vi "RunTest.vi"(8 "error in":errorcluster, 11 "Prueba21 in":refnum<class "Prueba21.lvclass">) -> (0 "error out":errorcluster, 2 "Resultado":string, 3 "Prueba21 out":refnum<class "Prueba21.lvclass">)   [LabVIEW 2019, in "Prueba21.lvclass"]
uses:
  Prueba21.lvclass
  Prueba21.lvclass/Prueba21.ctl
  QMH/Message Queue/Enqueue Message (Single).vi
  <vilib>/Utility/error.llb/Error Cluster From Error Code.vi
  RerenceAllControlsToolkit/_get mutiple control reference by name.vi
  RerenceAllControlsToolkit/_get control reference by name.vi
  <vilib>/ErrorRing/Error Ring.xnode
  QMH/Message Queue/Message Queue.lvlib
  QMH/User Event - Stop/User Event - Stop.lvlib
  Prueba/Prueba.lvclass
panel:
  out "TD":dbl
  out "Frecuencia":dbl
  out "voltaje":dbl
  in  "generar_ext":bool
  in  "Tab Control":enum32{"D1", "D2"}(tab)
  in  "CapturaGlobal_D1":bool
  in  "3_D1":bool
  in  "2_D1":bool
  out "LedVerdeD1":bool=TRUE
  in  "1_D1":bool
  out "LedRojoD1":bool=TRUE
  in  "Capturar_D1":bool
  out "Tabla_Referencia":string[][](table)
  out "grafica_frec_1":cluster{"f0":dbl, "df":dbl, "magnitude":dbl[]}[](graph) caption="Presion Sonora Vs Frencuencia"
  out "grafica_tiempo_1":waveform(dbl)[](graph) caption="Presion Sonora Vs Tiempo"
  in  "seguir_D2":bool
  in  "Capturar_D2":bool
  out "LedRojoD2":bool=TRUE
  out "LedVerdeD2":bool=TRUE
  in  "1_D2":bool
  in  "2_D2":bool
  in  "3_D2":bool
  out "Tabla_Presion_Sonora":string[][](table)
  out "Tabla_Frecuencia":string[][](table)
  out "Tabla_Distorsion_Total":string[][](table)
  out "grafica_frec_2":cluster{"f0":dbl, "df":dbl, "magnitude":dbl[]}[](graph) caption="Presion Sonora Vs Frencuencia"
  out "grafica_tiempo_2":waveform(dbl)[](graph) caption="Presion Sonora Vs Tiempo."
  in  "CapturaGlobal_D2":bool
  out "cumple":bool
  out "no_cumple":bool
  in  "salir":bool
  # "Captura Individual"
  # "21. Medición Nivel de Presión Sonora Calibrador Patrón"
  # "Nivel de Presión Sonora"
  # "Frecuencia"
  # "Distorsión Total (TD)"
  # "Captura Individual"
  # "Cumple"
  # "No Cumple"
  # "21. Medición Nivel de Presión Sonora Calibrador Patrón"
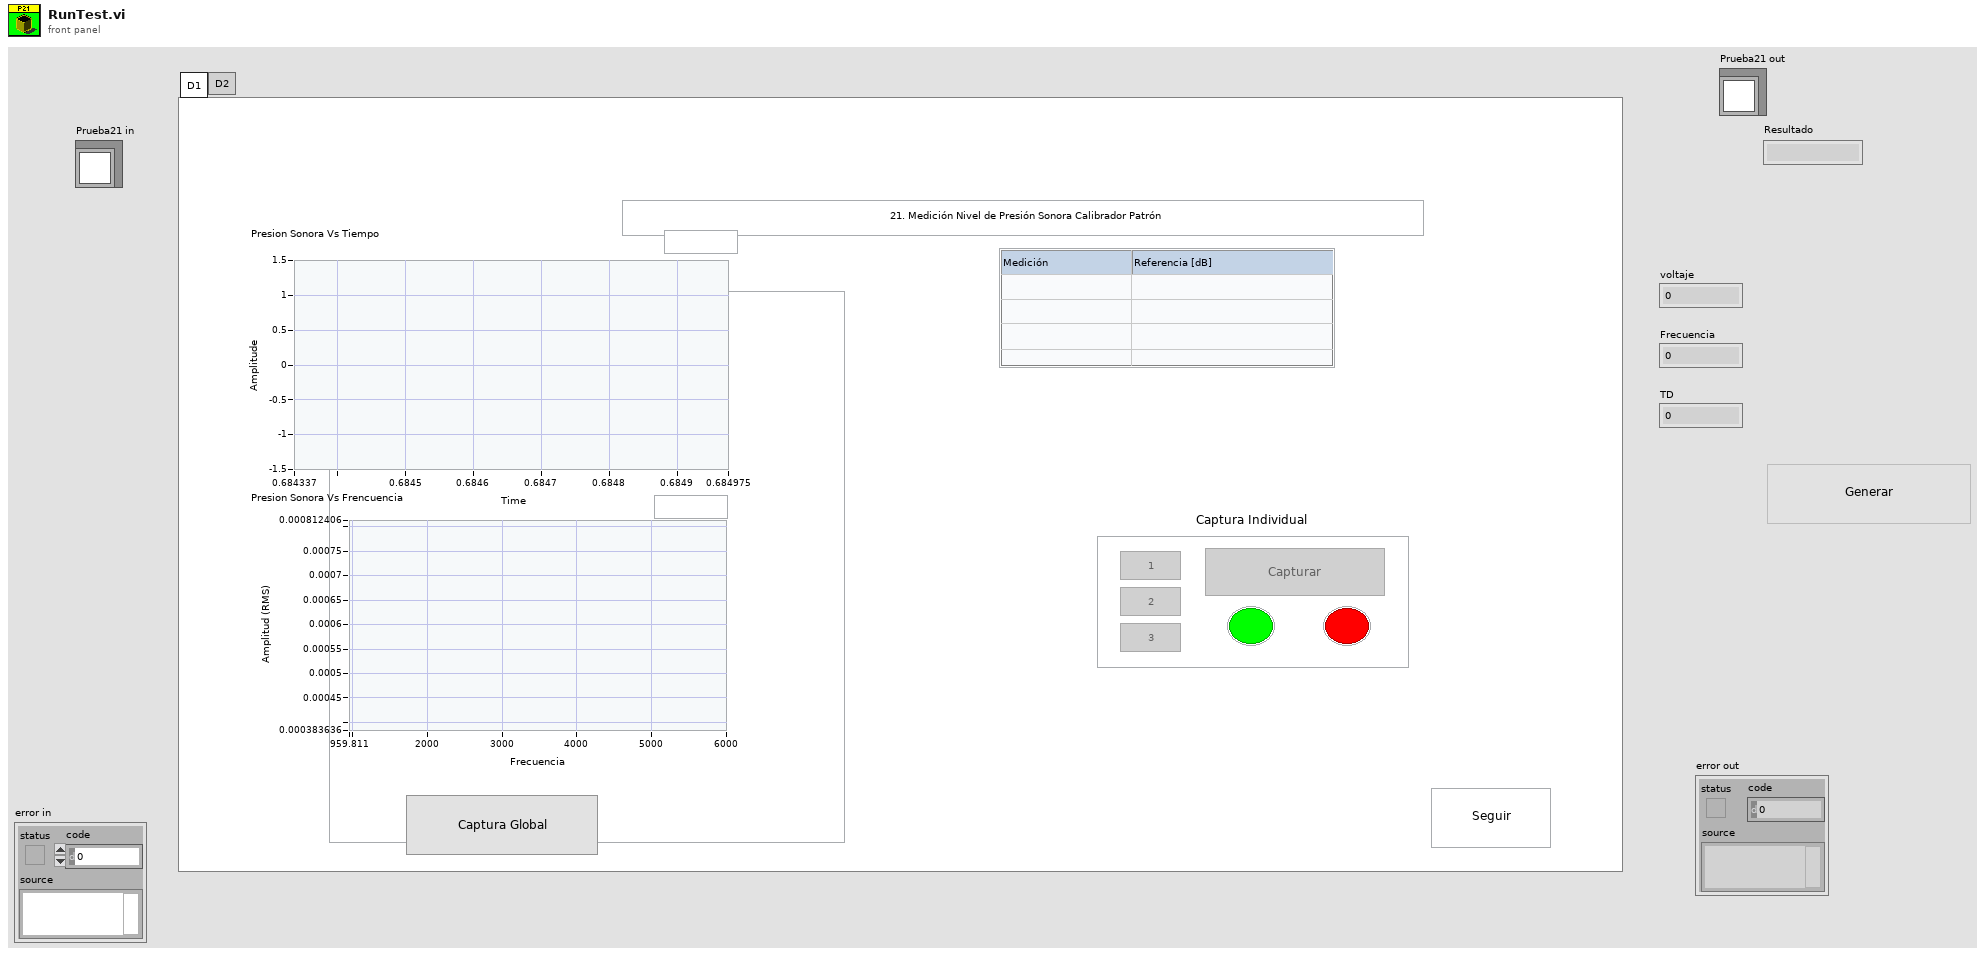
[diagram p1: front panel]
types:
  T1 = typedef "Message Queue.lvlib/All Message Queues.ctl" = cluster{"MHL":refnum<queue>, "Inst_CNT90":refnum<queue>, "Inst_DS360":refnum<queue>, "Inst_Keithley2002":refnum<queue>, "Inst_DAQ":refnum<queue>, "BD":refnum<queue>, "Pistofono":refnum<queue>, "Nexus":refnum<queue>}
  T2 = cluster{"ControlName":string, "ControlReference":refnum<vi>}[]
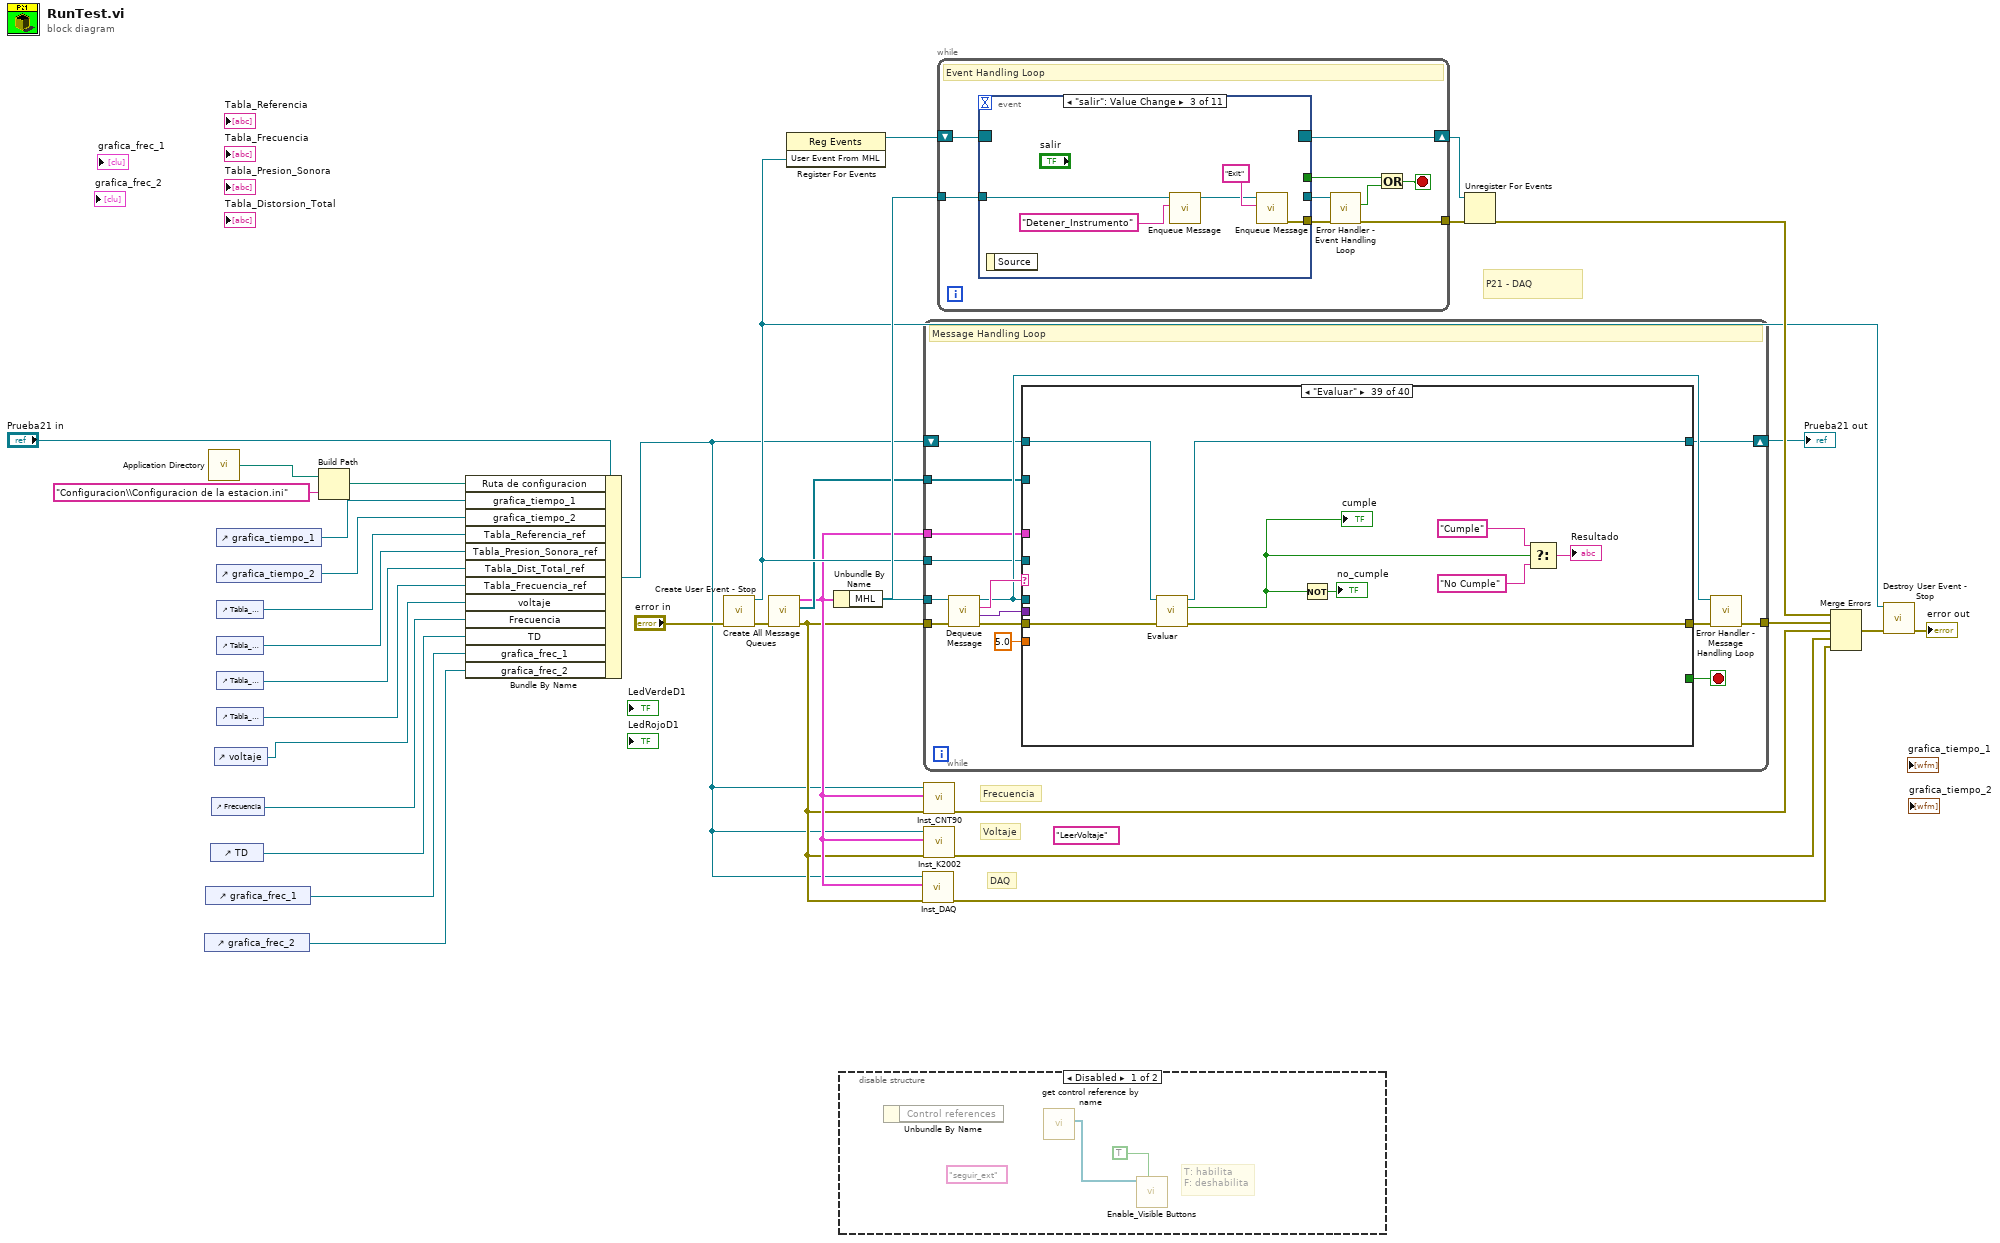
[diagram p0: block diagram]
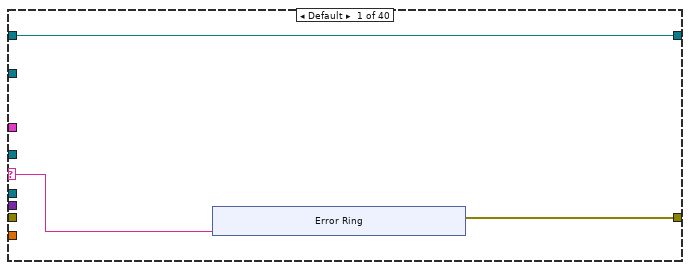
[diagram p3: hidden frame]
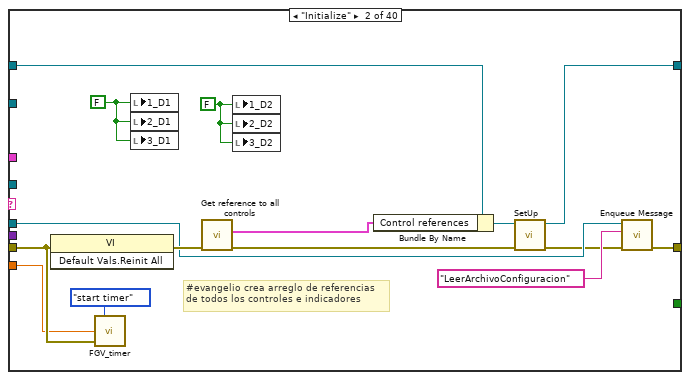
[diagram p4: hidden frame]
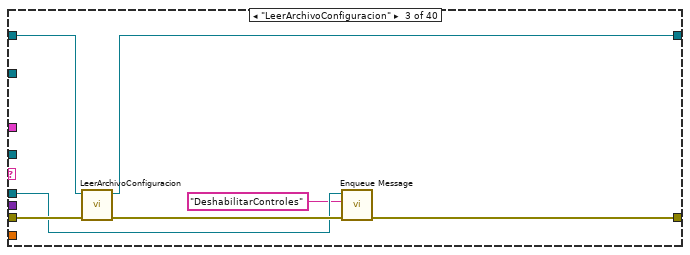
[diagram p5: hidden frame]
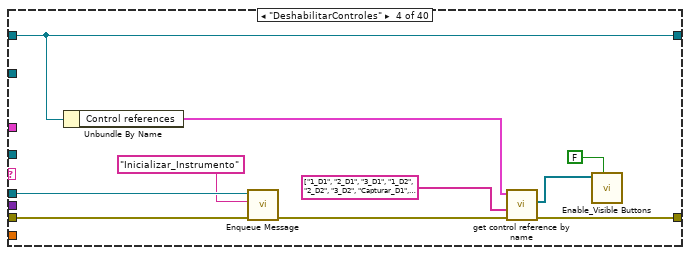
[diagram p6: hidden frame]
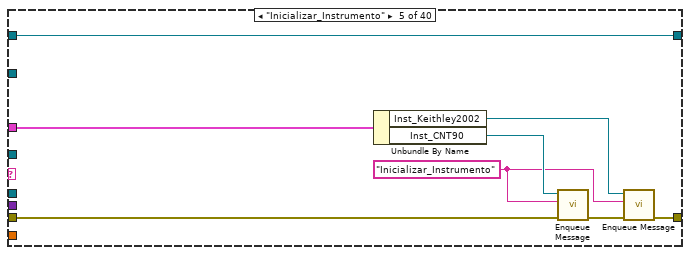
[diagram p7: hidden frame]
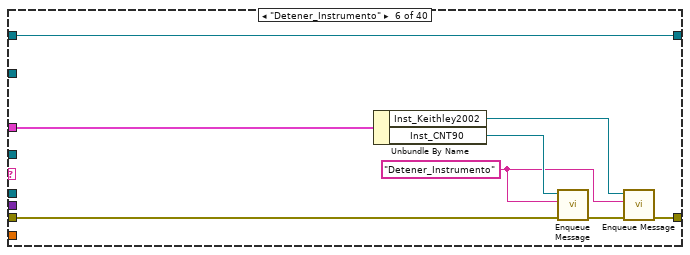
[diagram p8: hidden frame]
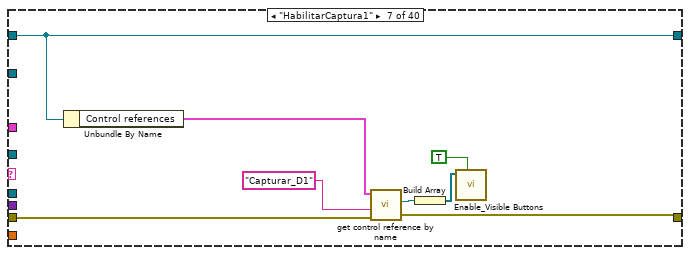
[diagram p9: hidden frame]
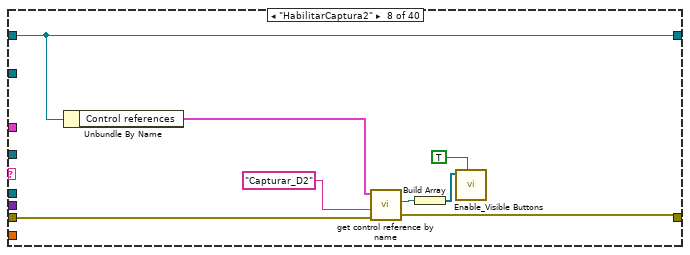
[diagram p10: hidden frame]
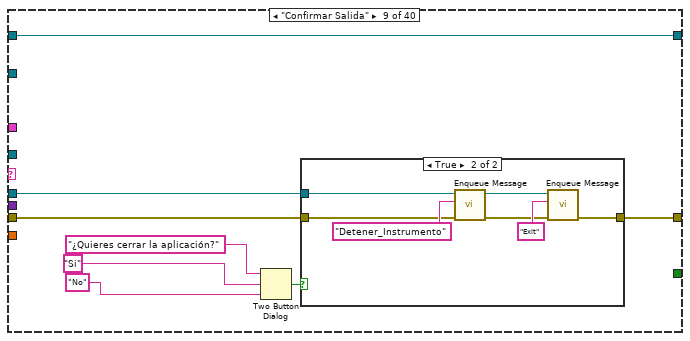
[diagram p11: hidden frame]
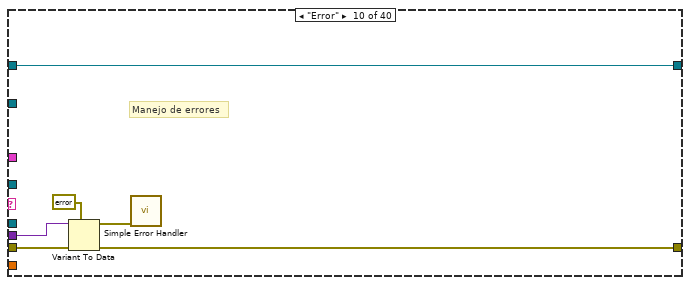
[diagram p13: hidden frame]
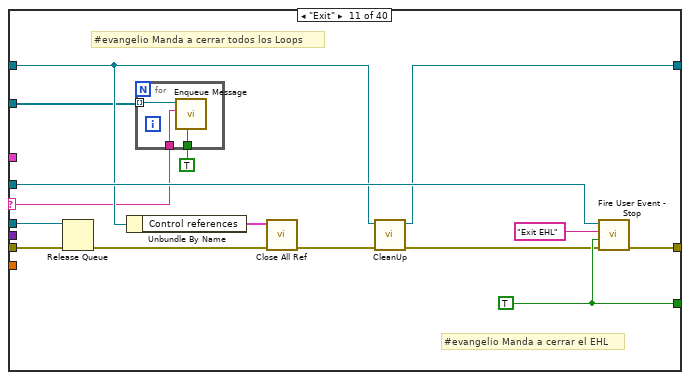
[diagram p14: hidden frame]
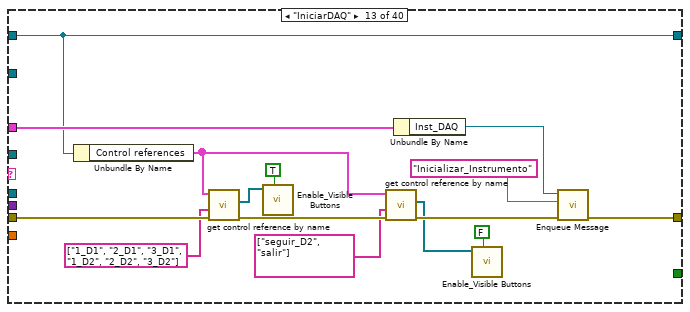
[diagram p16: hidden frame]
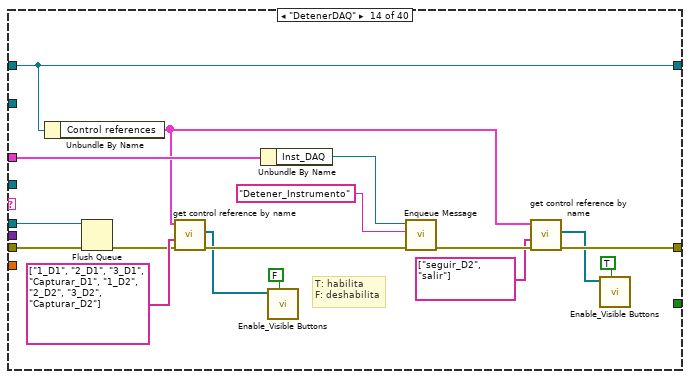
[diagram p17: hidden frame]
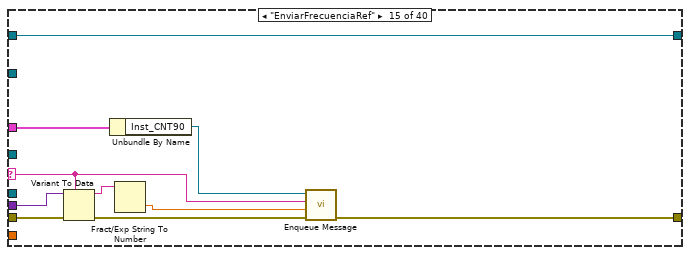
[diagram p18: hidden frame]
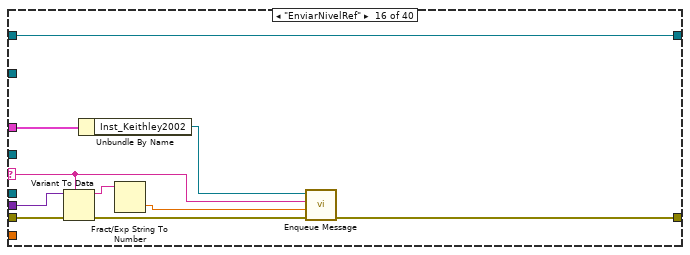
[diagram p19: hidden frame]
diagram:
  (unwired) "LeerVoltaje" ("Message")
  # "P21 - DAQ"
  # "DAQ"
  # "Voltaje"
  # "Frecuencia"
  n1 = control-ref of="grafica_frec_2"() -> (w1:refnum<vi>)
  n2 = control-ref of="grafica_frec_1"() -> (w2:refnum<vi>)
  n3 = call <vilib>:"Application Directory.vi"() -> ("Application Directory"=w19:path)
  n4 = control-ref of="TD"() -> (w3:refnum<vi>)
  n5 = control-ref of="Frecuencia"() -> (w4:refnum<vi>)
  n6 = control-ref of="voltaje"() -> (w5:refnum<vi>)
  n7 = control-ref of="grafica_tiempo_1"() -> (w12:refnum<vi>)
  n8 = control-ref of="grafica_tiempo_2"() -> (w11:refnum<vi>)
  n9 = control-ref of="Tabla_Referencia"() -> (w9:refnum<vi>)
  n10 = control-ref of="Tabla_Presion_Sonora"() -> (w8:refnum<vi>)
  n11 = control-ref of="Tabla_Distorsion_Total"() -> (w7:refnum<vi>)
  n12 = control-ref of="Tabla_Frecuencia"() -> (w6:refnum<vi>)
  n13 = Build Path(base path=w19, name or relative path="Configuracion\\Configuracion de la estacion.ini") -> (appended path=w18:path)
  n14 = Bundle By Name(cluster="Prueba21 in", "Ruta de configuracion"=w18, "grafica_tiempo_1"=w12, "grafica_tiempo_2"=w11, "Tabla_Referencia_ref"=w9, "Tabla_Presion_Sonora_ref"=w8, "Tabla_Dist_Total_ref"=w7, "Tabla_Frecuencia_ref"=w6, "voltaje"=w5, "Frecuencia"=w4, "TD"=w3, "grafica_frec_1"=w2, "grafica_frec_2"=w1) -> (w10:refnum<class "Prueba21.lvclass">)
  n15 = call "Create User Event - Stop.vi"("error in (no error)"="error in") -> ("error out"=w31:errorcluster, "User Event From MHL"=w25:refnum<user-event>)  [unwired: 9 in]
  n16 = call "Create All Message Queues.vi"("error in (no error)"=w31) -> ("error out"=w14:errorcluster, "PL Queues Array"=w16:refnum<queue>[], "All Message Queues out"=w15:T1)  [unwired: 8 in]
  n17 = register-events(w25) -> (reference out=w34:refnum<event-registration>)  [unwired: 2 in, 1 out]
  n18 = Unbundle By Name(w15) -> ("MHL"=w30:refnum<queue>)
  n19 = disable-structure shown="Disabled" {
    frame Disabled {
      (unwired) "seguir_ext" ("Control name")
      # "T: habilita\nF: deshabilita"
      n20 = Unbundle By Name() -> ("Control references"=w35)  [unwired: 1 in]
      n21 = call-poly "get control reference by name.vi"() -> ("error out"=w37:errorcluster, "References"=w36:refnum<vi>[], "Control names"=w39:string[])  [unwired: 5 in]
      n22 = call "Enable_Visible Buttons.vi"("Enable? (T)"=TRUE, "Controls Ref Array"=w36) -> ()  [unwired: 10 in]
    }
    frame Enabled {
    }
  }
  n23 = call "Inst_DAQ.vi"("error in"=w14, "All Message Queues in"=w15, "Prueba31 in"=w10) -> ("error out"=w13:errorcluster)  [unwired: 8 in]
  n24 = while {
    tunnel: w14 -> [w54]
    tunnel: w30 -> [w53]
    tunnel: [w47] -> w28
    shift-right: [w45] -> w26
    shift-left: w10 -> [w46]
    tunnel: w15 -> [w43]
    tunnel: w25 -> [w42]
    tunnel: w16 -> [w41]
    stop <- w44 stop-if-true
    # "Message Handling Loop"
    n25 = call "Dequeue Message.vi"("error in (no error)"=w54, "Message Queue"=w53) -> ("error out"=w50:errorcluster, "Message Data"=w51:variant, "Message"=w52:string, "dup Message Queue"=w49:refnum<queue>)  [unwired: 6 in]
    n26 = case shown="\"Evaluar\"" w52 {
      selector: w52 -> [w56 _ _ _ _ _ _ _ _ _ w153 _ _ _ w201 w211 _ _ _ _ _ _ _ _ _ _ _ _ _ _ _ _ _ _ _ _ _ _ _ _]
      tunnel: w49 -> [_ w76 w81 w88 _ _ _ _ w129 _ w164 _ _ w190 _ _ _ _ _ _ w254 w263 w283 w318 w332 _ _ _ _ _ w392 w403 w416 w436 w459 _ w469 _ _ _]
      tunnel: w51 -> [_ _ _ _ _ _ _ _ _ w146 _ _ _ _ w208 w218 _ _ _ _ _ _ _ _ _ _ _ _ _ _ _ _ _ w441 _ _ _ _ _ _]
      tunnel: w50 -> [_ w71 w86 w95 w97 w105 w119 w127 w135 w147 w163 w170 w178 w195 w209 w219 w222 w224 w239 w250 w259 w271 w290 w326 w335 w343 w360 w362 w377 w388 w397 w408 w424 w442 w461 w467 w478 w486 w500 w502]
      tunnel: [w55 w77 w82 w93 w99 w107 w117 w125 w134 w148 w161 w170 w175 w189 w205 w215 w222 w224 w236 w246 w257 w268 w288 w325 w334 w349 w357 w362 w374 w384 w395 w406 w421 w437 w444 w467 w470 w482 w499 w502] -> w48
      tunnel: w46 -> [w57 w78 w85 w94 w98 w106 w118 w126 w136 w150 w154 w169 w180 w196 w210 w220 w221 w223 w240 w251 w262 w267 w286 w323 w331 w342 w356 w361 w378 w389 w400 w411 w420 w439 w450 w466 w476 w484 w498 w501]
      tunnel: [w57 w66 w84 w94 w98 w106 w118 w126 w136 w150 w155 w169 w180 w196 w210 w220 w221 w223 w240 w251 w262 w265 w287 w324 w333 w342 w355 w361 w378 w389 w400 w411 w418 w439 w450 w466 w471 w483 w497 w501] -> w45
      tunnel: [_ _ _ _ _ _ _ _ _ _ w158 _ _ _ _ _ _ _ _ _ _ _ _ _ _ _ _ _ _ _ _ _ _ _ _ _ _ _ _ _] -> w44
      tunnel: w43 -> [_ _ _ _ w104 w112 _ _ _ _ _ _ w184 w200 w203 w213 _ _ w242 w245 w261 _ _ _ _ _ _ _ w380 w383 w399 w410 _ _ _ _ _ w481 _ _]
      tunnel: w42 -> [_ _ _ _ _ _ _ _ _ _ w160 _ _ _ _ _ _ _ _ _ _ _ _ _ _ _ _ _ _ _ _ _ _ _ _ _ _ _ _ _]
      tunnel: w41 -> [_ _ _ _ _ _ _ _ _ _ w151 _ _ _ _ _ _ _ _ _ _ _ _ _ _ _ _ _ _ _ _ _ _ _ _ _ _ _ _ _]
      tunnel: 5.0 ("time target") -> [_ w69 _ _ _ _ _ _ _ _ _ _ _ _ _ _ _ _ _ w248 _ w272 _ _ _ w348 _ _ _ w386 _ _ w425 _ w443 _ _ _ _ _]
      frame Default {
        n27 = xnode "Error Ring"("parameter 0"=w56) -> ("error out"=w55:errorcluster)
      }
      frame "Initialize" {
        w72 = FALSE ("1_D2")
        w73 = FALSE ("1_D1")
        # "#evangelio crea arreglo de referencias\nde todos los controles e indicadores"
        n28 = invoke class="VI" method="Default Vals.Reinit All"(error in=w71) -> (error out=w79:errorcluster)  [unwired: 2 in, 2 out]
        n29 = call "FGV_timer.vi"("error in (no error)"=w71, "time target"=w69, "action"=enum16{"get time", "start timer"}."start timer") -> ()  [unwired: 3 out]
        n30 = local write "1_D1"(w73) -> ()
        n31 = local write "2_D1"(w73) -> ()
        n32 = local write "3_D1"(w73) -> ()
        n33 = call "Get reference to all controls.vi"("error in (no error)"=w79) -> ("error out"=w67:errorcluster, "Control references"=w74:T2)  [unwired: 5 in]
        n34 = local write "1_D2"(w72) -> ()
        n35 = local write "2_D2"(w72) -> ()
        n36 = local write "3_D2"(w72) -> ()
        n37 = Bundle By Name(cluster=w78, "Control references"=w74) -> (w68:refnum<class "Prueba21.lvclass">)
        n38 = call-dynamic "SetUp.vi"("error in (no error)"=w67, "Prueba21 in"=w68) -> ("error out"=w65:errorcluster, "Prueba21 out"=w66:refnum<class "Prueba21.lvclass">)  [unwired: 8 in]
        n39 = call-poly "Enqueue Message.vi"("error in (no error)"=w65, "Message"="LeerArchivoConfiguracion", "Message Queue"=w76) -> ("error out"=w77:errorcluster)  [unwired: 7 in, 1 out]
      }
      frame "LeerArchivoConfiguracion" {
        n40 = call "LeerArchivoConfiguracion.vi"("error in"=w86, "Prueba31 in"=w85) -> ("error out"=w83:errorcluster, "Prueba31 out"=w84:refnum<class "Prueba21.lvclass">)  [unwired: 8 in]
        n41 = call-poly "Enqueue Message.vi"("error in (no error)"=w83, "Message"="DeshabilitarControles", "Message Queue"=w81) -> ("error out"=w82:errorcluster)  [unwired: 7 in, 1 out]
      }
      frame "DeshabilitarControles" {
        n42 = Unbundle By Name(w94) -> ("Control references"=w96:T2)
        n43 = call-poly "Enqueue Message.vi"("error in (no error)"=w95, "Message"="Inicializar_Instrumento", "Message Queue"=w88) -> ("error out"=w89:errorcluster)  [unwired: 7 in, 1 out]
        n44 = call-poly "get control reference by name.vi"("error in (no error)"=w89, "Control names"=string[] ["1_D1", "2_D1", "3_D1", "1_D2", "2_D2", "3_D2", "Capturar_D1", "Capturar_D2"], "Control references"=w96) -> ("error out"=w93:errorcluster, "References"=w91:refnum<vi>[])  [unwired: 3 in]
        n45 = call "Enable_Visible Buttons.vi"("Enable? (T)"=FALSE, "Controls Ref Array"=w91) -> ()  [unwired: 10 in]
      }
      frame "Inicializar_Instrumento" {
        w100 = "Inicializar_Instrumento" ("Message")
        n46 = Unbundle By Name(w104) -> ("Inst_Keithley2002"=w101:refnum<queue>, "Inst_CNT90"=w103:refnum<queue>)
        n47 = call-poly "Enqueue Message.vi"("error in (no error)"=w97, "Message"=w100, "Message Queue"=w103) -> ("error out"=w102:errorcluster)  [unwired: 7 in, 1 out]
        n48 = call-poly "Enqueue Message.vi"("error in (no error)"=w102, "Message"=w100, "Message Queue"=w101) -> ("error out"=w99:errorcluster)  [unwired: 7 in, 1 out]
      }
      frame "Detener_Instrumento" {
        w108 = "Detener_Instrumento" ("Message")
        n49 = Unbundle By Name(w112) -> ("Inst_Keithley2002"=w109:refnum<queue>, "Inst_CNT90"=w111:refnum<queue>)
        n50 = call-poly "Enqueue Message.vi"("error in (no error)"=w105, "Message"=w108, "Message Queue"=w111) -> ("error out"=w110:errorcluster)  [unwired: 7 in, 1 out]
        n51 = call-poly "Enqueue Message.vi"("error in (no error)"=w110, "Message"=w108, "Message Queue"=w109) -> ("error out"=w107:errorcluster)  [unwired: 7 in, 1 out]
      }
      frame "HabilitarCaptura1" {
        n52 = Unbundle By Name(w118) -> ("Control references"=w120:T2)
        n53 = call-poly "get control reference by name.vi"("error in (no error)"=w119, "Control name"="Capturar_D1", "Control references"=w120) -> ("error out"=w117:errorcluster, "Ctl Refnum"=w114:refnum<vi>)  [unwired: 3 in]
        n54 = Build Array(w114) -> (w113:refnum<vi>[])
        n55 = call "Enable_Visible Buttons.vi"("Enable? (T)"=TRUE, "Controls Ref Array"=w113) -> ()  [unwired: 10 in]
      }
      frame "HabilitarCaptura2" {
        n56 = Unbundle By Name(w126) -> ("Control references"=w128:T2)
        n57 = call-poly "get control reference by name.vi"("error in (no error)"=w127, "Control name"="Capturar_D2", "Control references"=w128) -> ("error out"=w125:errorcluster, "Ctl Refnum"=w122:refnum<vi>)  [unwired: 3 in]
        n58 = Build Array(w122) -> (w121:refnum<vi>[])
        n59 = call "Enable_Visible Buttons.vi"("Enable? (T)"=TRUE, "Controls Ref Array"=w121) -> ()  [unwired: 10 in]
      }
      frame "Confirmar Salida" {
        n60 = Two Button Dialog(message="¿Quieres cerrar la aplicación?", 1:"No" ("T button name (\"OK\")"), 2:"Si" ("T button name (\"OK\")")) -> (T button?=w130:bool)
        n61 = case shown="True" w130 {
          tunnel: w135 -> [w137 w140]
          tunnel: [w137 w144] -> w134
          tunnel: w129 -> [_ w141]
          frame False {
          }
          frame True {
            n62 = call-poly "Enqueue Message.vi"("error in (no error)"=w140, "Message"="Detener_Instrumento", "Message Queue"=w141) -> ("error out"=w139:errorcluster, "dup Message Queue"=w138:refnum<queue>)  [unwired: 7 in]
            n63 = call-poly "Enqueue Message.vi"("error in (no error)"=w139, "Message"="Exit", "Message Queue"=w138) -> ("error out"=w144:errorcluster)  [unwired: 7 in, 1 out]
          }
        }
      }
      frame "Error" {
        # "Manejo de errores"
        n64 = Variant To Data(error in=w147, type=errorcluster {"status"=FALSE, "code"=0, "source"=""} ("error constant"), Variant=w146) -> (data=w145:errorcluster, error out=w148:errorcluster)
        n65 = call <vilib>:"Simple Error Handler.vi"("error in (no error)"=w145) -> ()  [unwired: 4 in, 5 out]
      }
      frame "Exit" {
        w158 = TRUE
        # "#evangelio Manda a cerrar el EHL"
        # "#evangelio Manda a cerrar todos los Loops"
        n66 = Release Queue(queue=w164, error in (no error)=w163) -> (error out=w162:errorcluster)  [unwired: 1 in, 2 out]
        n67 = Unbundle By Name(w154) -> ("Control references"=w165:T2)
        n68 = for {
          tunnel: w151 -> [w168] mode=indexing
          tunnel: w153 -> [w167]
          tunnel: TRUE -> [w166]
          n69 = call-poly "Enqueue Message.vi"("Priority Message? (F)"=w166, "Message"=w167, "Message Queue"=w168) -> ()  [unwired: 7 in, 2 out]
        }
        n70 = call "Close All Ref.vi"("error in (no error)"=w162, "Control references"=w165) -> ("error out"=w157:errorcluster)  [unwired: 9 in]
        n71 = call-dynamic "CleanUp.vi"("error in (no error)"=w157, "Prueba21 in"=w154) -> ("error out"=w156:errorcluster, "Prueba21 out"=w155:refnum<class "Prueba21.lvclass">)  [unwired: 8 in]
        n72 = call "Fire User Event - Stop.vi"("error in (no error)"=w156, "Event Data"=w158, "User Event"="Exit EHL", "User Event in"=w160) -> ("error out"=w161:errorcluster)  [unwired: 7 in]
      }
      frame "---- Captura Global  ----" {
      }
      frame "IniciarDAQ" {
        n73 = Unbundle By Name(w180) -> ("Control references"=w174:T2)
        n74 = call-poly "get control reference by name.vi"("error in (no error)"=w178, "Control names"=string[] ["1_D1", "2_D1", "3_D1", "1_D2", "2_D2", "3_D2"] ("Control name"), "Control references"=w174) -> ("error out"=w179:errorcluster, "References"=w181:refnum<vi>[])  [unwired: 3 in]
        n75 = call "Enable_Visible Buttons.vi"("Enable? (T)"=TRUE, "Controls Ref Array"=w181) -> ()  [unwired: 10 in]
        n76 = call-poly "get control reference by name.vi"("Control names"=string[] ["seguir_D2", "salir"] ("Message"), "Control references"=w174) -> ("References"=w172:refnum<vi>[])  [unwired: 4 in, 1 out]
        n77 = Unbundle By Name(w184) -> ("Inst_DAQ"=w183:refnum<queue>)
        n78 = call "Enable_Visible Buttons.vi"("Enable? (T)"=FALSE, "Controls Ref Array"=w172) -> ()  [unwired: 10 in]
        n79 = call-poly "Enqueue Message.vi"("error in (no error)"=w179, "Message"="Inicializar_Instrumento", "Message Queue"=w183) -> ("error out"=w175:errorcluster)  [unwired: 7 in, 1 out]
      }
      frame "DetenerDAQ" {
        # "T: habilita\nF: deshabilita"
        n80 = Unbundle By Name(w196) -> ("Control references"=w188:T2)
        n81 = Flush Queue(queue=w190, error in (no error)=w195) -> (error out=w191:errorcluster)  [unwired: 2 out]
        n82 = call-poly "get control reference by name.vi"("error in (no error)"=w191, "Control names"=string[] ["1_D1", "2_D1", "3_D1", "Capturar_D1", "1_D2", "2_D2", "3_D2", "Capturar_D2"] ("Control name"), "Control references"=w188) -> ("error out"=w194:errorcluster, "References"=w192:refnum<vi>[])  [unwired: 3 in]
        n83 = Unbundle By Name(w200) -> ("Inst_DAQ"=w199:refnum<queue>)
        n84 = call "Enable_Visible Buttons.vi"("Enable? (T)"=FALSE, "Controls Ref Array"=w192) -> ()  [unwired: 10 in]
        n85 = call-poly "Enqueue Message.vi"("error in (no error)"=w194, "Message"="Detener_Instrumento", "Message Queue"=w199) -> ("error out"=w189:errorcluster)  [unwired: 7 in, 1 out]
        n86 = call-poly "get control reference by name.vi"("Control names"=string[] ["seguir_D2", "salir"] ("Message"), "Control references"=w188) -> ("References"=w186:refnum<vi>[])  [unwired: 4 in, 1 out]
        n87 = call "Enable_Visible Buttons.vi"("Enable? (T)"=TRUE, "Controls Ref Array"=w186) -> ()  [unwired: 10 in]
      }
      frame "EnviarFrecuenciaRef" {
        n88 = Variant To Data(error in=w209, type=w201, Variant=w208) -> (data=w207:string, error out=w206:errorcluster)
        n89 = Unbundle By Name(w203) -> ("Inst_CNT90"=w202:refnum<queue>)
        n90 = Fract/Exp String To Number(string=w207) -> (number=w204:dbl)  [unwired: 3 in, 1 out]
        n91 = call-poly "Enqueue Message.vi"("error in (no error)"=w206, "Message Data"=w204, "Message"=w201, "Message Queue"=w202) -> ("error out"=w205:errorcluster)  [unwired: 6 in, 1 out]
      }
      frame "EnviarNivelRef" {
        n92 = Variant To Data(error in=w219, type=w211, Variant=w218) -> (data=w217:string, error out=w216:errorcluster)
        n93 = Unbundle By Name(w213) -> ("Inst_Keithley2002"=w212:refnum<queue>)
        n94 = Fract/Exp String To Number(string=w217) -> (number=w214:dbl)  [unwired: 3 in, 1 out]
        n95 = call-poly "Enqueue Message.vi"("error in (no error)"=w216, "Message Data"=w214, "Message"=w211, "Message Queue"=w212) -> ("error out"=w215:errorcluster)  [unwired: 6 in, 1 out]
      }
      frame "Evaluacion_Ext" {
        # "como32"
        # "Crear SubVI de evaluacion"
      }
      frame "---- Captura 1 ----" {
      }
      frame "IniciarCaptura1" {
        # "T: habilita\nF: deshabilita"
        n96 = Unbundle By Name(w240) -> ("Control references"=w230:T2)
        n97 = call-poly "get control reference by name.vi"("error in (no error)"=w239, "Control names"=string[] ["1_D1", "2_D1", "3_D1"] ("Control name"), "Control references"=w230) -> ("error out"=w231:errorcluster, "References"=w241:refnum<vi>[])  [unwired: 3 in]
        n98 = call "Enable_Visible Buttons.vi"("Enable? (T)"=TRUE, "Controls Ref Array"=w241) -> ()  [unwired: 10 in]
        n99 = Unbundle By Name(w242) -> ("MHL"=w235:refnum<queue>)
        n100 = call-poly "get control reference by name.vi"("error in (no error)"=w231, "Control name"="CapturaGlobal_D1" ("Message"), "Control references"=w230) -> ("error out"=w225:errorcluster, "Ctl Refnum"=w227:refnum<vi>)  [unwired: 3 in]
        n101 = Build Array(w227) -> (w226:refnum<vi>[])
        n102 = call "Enable_Visible Buttons.vi"("Enable? (T)"=FALSE, "Controls Ref Array"=w226) -> ()  [unwired: 10 in]
        n103 = local write "LedVerdeD1"(TRUE ("LedVerdeD1")) -> ()
        n104 = local write "LedRojoD1"(FALSE ("LedRojoD1")) -> ()
        n105 = call-poly "Enqueue Message.vi"("error in (no error)"=w225, "Message"="IniciarTimer", "Message Queue"=w235) -> ("error out"=w236:errorcluster)  [unwired: 7 in, 1 out]
      }
      frame "IniciarTimer" {
        n106 = Unbundle By Name(w245) -> ("MHL"=w244:refnum<queue>)
        n107 = call "FGV_timer.vi"("error in (no error)"=w250, "time target"=w248, "action"=enum16{"get time", "start timer"}."start timer") -> ("error out"=w247:errorcluster)  [unwired: 2 out]
        n108 = call-poly "Enqueue Message.vi"("error in (no error)"=w247, "Message"="Leer_Voltaje", "Message Queue"=w244) -> ("error out"=w246:errorcluster)  [unwired: 7 in, 1 out]
      }
      frame "Leer_Voltaje" {
        n109 = Unbundle By Name(w261) -> ("Inst_Keithley2002"=w260:refnum<queue>)
        n110 = call-poly "Enqueue Message.vi"("error in (no error)"=w259, "Message"="Leer_Instrumento", "Message Queue"=w260) -> ("error out"=w256:errorcluster)  [unwired: 7 in, 1 out]
        n111 = call "Time Delay"("error in (no error)"=w256, "Delay Time (s)"=0.5) -> ("error out"=w253:errorcluster)  [unwired: 9 in]
        n112 = call-poly "Enqueue Message.vi"("error in (no error)"=w253, "Message"="Leer_Indicador_V", "Message Queue"=w254) -> ("error out"=w257:errorcluster)  [unwired: 7 in, 1 out]
      }
      frame "Leer_Indicador_V" {
        n113 = Unbundle By Name(w267) -> ("voltaje"=w266:refnum<vi>)
        n114 = property class="DigNum (strict)"(reference=w266) -> ("Value"=w264:dbl)  [unwired: 1 in, 2 out]
        n115 = call "FGV_timer.vi"("error in (no error)"=w271, "time target"=w272, "action"=enum16{"get time", "start timer"}."get time") -> ("error out"=w269:errorcluster, "time elapsed?"=w270:bool)  [unwired: 1 out]
        n116 = Bundle By Name(cluster=w267, "voltaje"=w264) -> (w265:refnum<class "Prueba21.lvclass">)
        n117 = case shown="True" w270 {
          tunnel: w269 -> [w276 w280]
          tunnel: [w275 w279] -> w268
          tunnel: w263 -> [w274 w278]
          frame True {
            n118 = call-poly "Enqueue Message.vi"("error in (no error)"=w276, "Message"="CalcularDB_Ref", "Message Queue"=w274) -> ("error out"=w275:errorcluster)  [unwired: 7 in, 1 out]
          }
          frame False {
            n119 = call-poly "Enqueue Message.vi"("error in (no error)"=w280, "Message"="Leer_Voltaje", "Message Queue"=w278) -> ("error out"=w279:errorcluster)  [unwired: 7 in, 1 out]
          }
        }
      }
      frame "CalcularDB_Ref" {
        n120 = Flush Queue(queue=w283, error in (no error)=w290) -> (queue out=w282:refnum<queue>, error out=w284:errorcluster)  [unwired: 1 out]
        n121 = Unbundle By Name(w286) -> ("voltaje"=w285:dbl)
        "voltaje" <- w285
        n122 = local read "Tab Control"() -> (w289:enum32{"D1", "D2"})
        n123 = case shown="\"D2\"" w289 {
          tunnel: w284 -> [w297 w304]
          tunnel: w285 -> [w298 w301]
          tunnel: w286 -> [w299 w302]
          tunnel: [w295 w306] -> w288
          tunnel: [w293 w300] -> w287
          tunnel: w282 -> [w294 w305]
          frame "D1", Default {
            n124 = call "ActualizarTablaReferencia.vi"("error in (no error)"=w297, "medido"=w298, "Prueba21_1"=w299) -> ("error out"=w296:errorcluster, "Prueba21_1"=w293:refnum<class "Prueba21.lvclass">)  [unwired: 7 in]
            n125 = Unbundle By Name(w293) -> ("Tabla_Referencia"=w292:string[][])
            n126 = local write "Tabla_Referencia"(w292) -> ()
            n127 = call-poly "Enqueue Message.vi"("error in (no error)"=w296, "Message"="DetenerCaptura1", "Message Queue"=w294) -> ("error out"=w295:errorcluster)  [unwired: 7 in, 1 out]
          }
          frame "D2" {
            n128 = call "ActualizarTablaNivelPresionSonora.vi"("error in (no error)"=w304, "medido"=w301, "Prueba21_1"=w302) -> ("error out"=w303:errorcluster, "Prueba21_1"=w300:refnum<class "Prueba21.lvclass">)  [unwired: 7 in]
            n129 = disable-structure shown="Enabled" {
              disable-tunnel: [w311 w314] -> w306
              disable-tunnel: w305 -> [w309 w313]
              disable-tunnel: w303 -> [w308 w315]
              frame Disabled {
                n130 = call-poly "Enqueue Message.vi"("error in (no error)"=w308, "Message"="DetenerCaptura2", "Message Queue"=w309) -> ("error out"=w311:errorcluster)  [unwired: 7 in, 1 out]
              }
              frame Enabled {
                n131 = call-poly "Enqueue Message.vi"("error in (no error)"=w315, "Message"="CalcularFrec", "Message Queue"=w313) -> ("error out"=w314:errorcluster)  [unwired: 7 in, 1 out]
              }
            }
            n132 = Unbundle By Name(w300) -> ("Tabla_Presion_Sonora"=w307:string[][])
            n133 = local write "Tabla_Presion_Sonora"(w307) -> ()
          }
        }
      }
      frame "CalcularFrec" {
        n134 = Flush Queue(queue=w318, error in (no error)=w326) -> (queue out=w317:refnum<queue>, error out=w319:errorcluster)  [unwired: 1 out]
        n135 = Unbundle By Name(w323) -> ("frecuencia"=w322:dbl)
        "Frecuencia" <- w322
        n136 = call "ActualizarTablaFrecuencia.vi"("error in (no error)"=w319, "medido"=w322, "Prueba21_1"=w323) -> ("error out"=w320:errorcluster, "Prueba21_1"=w324:refnum<class "Prueba21.lvclass">)  [unwired: 7 in]
        n137 = Unbundle By Name(w324) -> ("Tabla_Frecuencia"=w321:string[][])
        n138 = local write "Tabla_Frecuencia"(w321) -> ()
        n139 = call-poly "Enqueue Message.vi"("error in (no error)"=w320, "Message"="CalcularTD", "Message Queue"=w317) -> ("error out"=w325:errorcluster)  [unwired: 7 in, 1 out]
      }
      frame "CalcularTD" {
        n140 = Unbundle By Name(w331) -> ("TD"=w330:dbl)
        "TD" <- w330
        n141 = call "ActualizarTablaTD.vi"("error in (no error)"=w335, "medido"=w330, "Prueba21_1"=w331) -> ("error out"=w327:errorcluster, "Prueba21_1"=w333:refnum<class "Prueba21.lvclass">)  [unwired: 7 in]
        n142 = Unbundle By Name(w333) -> ("Tabla_Dist_Total"=w329:string[][])
        n143 = local write "Tabla_Distorsion_Total"(w329) -> ()
        n144 = call-poly "Enqueue Message.vi"("error in (no error)"=w327, "Message"="DetenerCaptura2", "Message Queue"=w332) -> ("error out"=w334:errorcluster)  [unwired: 7 in, 1 out]
      }
      frame "DetenerCaptura1" {
        w351 = FALSE ("Capturar_D1")
        # "Habikita Boton CapturaGlobalD1"
        # "Deshabilita Boton Captura 1"
        # "reinicia timer"
        n145 = Unbundle By Name(w342) -> ("Control references"=w337:T2)
        n146 = call-poly "get control reference by name.vi"("error in (no error)"=w343, "Control name"="Capturar_D1", "Control references"=w337) -> ("error out"=w338:errorcluster, "Ctl Refnum"=w345:refnum<vi>)  [unwired: 3 in]
        n147 = Build Array(w345) -> (w344:refnum<vi>[])
        n148 = call "Enable_Visible Buttons.vi"("Enable? (T)"=FALSE, "Controls Ref Array"=w344) -> ()  [unwired: 10 in]
        n149 = call-poly "get control reference by name.vi"("error in (no error)"=w338, "Control name"="CapturaGlobal_D1", "Control references"=w337) -> ("Ctl Refnum"=w340:refnum<vi>)  [unwired: 3 in, 1 out]
        n150 = Build Array(w340) -> (w341:refnum<vi>[])
        n151 = call "Enable_Visible Buttons.vi"("Enable? (T)"=TRUE, "Controls Ref Array"=w341) -> ()  [unwired: 10 in]
        n152 = local write "1_D1"(w351) -> ()
        n153 = local write "2_D1"(w351) -> ()
        n154 = local write "3_D1"(w351) -> ()
        n155 = call "FGV_timer.vi"("time target"=w348, "action"=enum16{"get time", "start timer"}."start timer") -> ("error out"=w349:errorcluster)  [unwired: 1 in, 2 out]
        n156 = local write "Capturar_D1"(FALSE ("Capturar_D1")) -> ()
        n157 = local write "LedVerdeD1"(FALSE ("LedVerdeD1")) -> ()
        n158 = local write "LedRojoD1"(TRUE ("LedRojoD1")) -> ()
      }
      frame "SeguirD2" {
        n159 = property on="Tab Control" class="TabCtl (strict)"(error in=w360, "Value"=enum32{"D1", "D2"}."D2" ("Tab Control")) -> (error out=w359:errorcluster)  [unwired: 1 in, 1 out]
        n160 = call "SacarNivelRefTablaRef.vi"("error in (no error)"=w359, "Prueba21 in"=w356) -> ("error out"=w357:errorcluster, "Prueba21 out"=w355:refnum<class "Prueba21.lvclass">)  [unwired: 8 in]
      }
      frame "---- Captura 2 ----" {
      }
      frame "IniciarCaptura2" {
        # "T: habilita\nF: deshabilita"
        n161 = Unbundle By Name(w378) -> ("Control references"=w364:T2)
        n162 = call-poly "get control reference by name.vi"("error in (no error)"=w377, "Control names"=string[] ["1_D2", "2_D2", "3_D2"] ("Control name"), "Control references"=w364) -> ("error out"=w365:errorcluster, "References"=w379:refnum<vi>[])  [unwired: 3 in]
        n163 = call "Enable_Visible Buttons.vi"("Enable? (T)"=TRUE, "Controls Ref Array"=w379) -> ()  [unwired: 10 in]
        n164 = Unbundle By Name(w380) -> ("MHL"=w373:refnum<queue>)
        n165 = call-poly "get control reference by name.vi"("error in (no error)"=w365, "Control name"="CapturaGlobal_D2" ("Message"), "Control references"=w364) -> ("error out"=w363:errorcluster, "Ctl Refnum"=w367:refnum<vi>)  [unwired: 3 in]
        n166 = Build Array(w367) -> (w366:refnum<vi>[])
        n167 = call "Enable_Visible Buttons.vi"("Enable? (T)"=FALSE, "Controls Ref Array"=w366) -> ()  [unwired: 10 in]
        n168 = local write "LedVerdeD2"(TRUE ("LedVerdeD1")) -> ()
        n169 = local write "LedRojoD2"(FALSE ("LedRojoD1")) -> ()
        n170 = call-poly "Enqueue Message.vi"("error in (no error)"=w363, "Message"="IniciarTimer_2", "Message Queue"=w373) -> ("error out"=w374:errorcluster)  [unwired: 7 in, 1 out]
      }
      frame "IniciarTimer_2" {
        n171 = Unbundle By Name(w383) -> ("MHL"=w382:refnum<queue>)
        n172 = call "FGV_timer.vi"("error in (no error)"=w388, "time target"=w386, "action"=enum16{"get time", "start timer"}."start timer") -> ("error out"=w385:errorcluster)  [unwired: 2 out]
        n173 = call-poly "Enqueue Message.vi"("error in (no error)"=w385, "Message"="Leer_Voltaje_2", "Message Queue"=w382) -> ("error out"=w384:errorcluster)  [unwired: 7 in, 1 out]
      }
      frame "Leer_Voltaje_2" {
        n174 = Unbundle By Name(w399) -> ("Inst_Keithley2002"=w398:refnum<queue>)
        n175 = call-poly "Enqueue Message.vi"("error in (no error)"=w397, "Message"="Leer_Instrumento", "Message Queue"=w398) -> ("error out"=w394:errorcluster)  [unwired: 7 in, 1 out]
        n176 = call "Time Delay2"("error in (no error)"=w394, "Delay Time (s)"=0.5) -> ("error out"=w391:errorcluster)  [unwired: 9 in]
        n177 = call-poly "Enqueue Message.vi"("error in (no error)"=w391, "Message"="Leer_Frecuencia_2", "Message Queue"=w392) -> ("error out"=w395:errorcluster)  [unwired: 7 in, 1 out]
      }
      frame "Leer_Frecuencia_2" {
        n178 = Unbundle By Name(w410) -> ("Inst_CNT90"=w409:refnum<queue>)
        n179 = call-poly "Enqueue Message.vi"("error in (no error)"=w408, "Message"="Leer_Instrumento", "Message Queue"=w409) -> ("error out"=w405:errorcluster)  [unwired: 7 in, 1 out]
        n180 = call "Time Delay3"("error in (no error)"=w405, "Delay Time (s)"=0.5) -> ("error out"=w402:errorcluster)  [unwired: 9 in]
        n181 = call-poly "Enqueue Message.vi"("error in (no error)"=w402, "Message"="Leer_Indicador_2", "Message Queue"=w403) -> ("error out"=w406:errorcluster)  [unwired: 7 in, 1 out]
      }
      frame "Leer_Indicador_2" {
        n182 = Unbundle By Name(w420) -> ("voltaje"=w419:refnum<vi>, "Frecuencia"=w415:refnum<vi>, "TD"=w413:refnum<vi>)
        n183 = property class="DigNum (strict)"(reference=w415) -> ("Value"=w414:dbl)  [unwired: 1 in, 2 out]
        n184 = property class="DigNum (strict)"(reference=w413) -> ("Value"=w412:dbl)  [unwired: 1 in, 2 out]
        n185 = property class="DigNum (strict)"(reference=w419) -> ("Value"=w417:dbl)  [unwired: 1 in, 2 out]
        n186 = call "FGV_timer.vi"("error in (no error)"=w424, "time target"=w425, "action"=enum16{"get time", "start timer"}."get time") -> ("error out"=w422:errorcluster, "time elapsed?"=w423:bool)  [unwired: 1 out]
        n187 = Bundle By Name(cluster=w420, "voltaje"=w417, "frecuencia"=w414, "TD"=w412) -> (w418:refnum<class "Prueba21.lvclass">)
        n188 = case shown="True" w423 {
          tunnel: w422 -> [w429 w433]
          tunnel: [w428 w432] -> w421
          tunnel: w416 -> [w427 w431]
          frame True {
            n189 = call-poly "Enqueue Message.vi"("error in (no error)"=w429, "Message"="CalcularDB_Ref", "Message Queue"=w427) -> ("error out"=w428:errorcluster)  [unwired: 7 in, 1 out]
          }
          frame False {
            n190 = call-poly "Enqueue Message.vi"("error in (no error)"=w433, "Message"="Leer_Voltaje_2", "Message Queue"=w431) -> ("error out"=w432:errorcluster)  [unwired: 7 in, 1 out]
          }
        }
      }
      frame "ActualizarOtrasTablas" {
        n191 = Variant To Data(error in=w442, type=dbl[] [] ("time target"), Variant=w441) -> (error out=w438:errorcluster)  [unwired: 1 out]
        n192 = call-poly "Enqueue Message.vi"("error in (no error)"=w438, "Message"="DetenerCaptura2", "Message Queue"=w436) -> ("error out"=w437:errorcluster)  [unwired: 7 in, 1 out]
      }
      frame "DetenerCaptura2" {
        w462 = FALSE ("Capturar_D1")
        # "reinicia timer"
        # "Deshabilita Boton Captura 2"
        n193 = local write "Capturar_D2"(FALSE ("Capturar_D1")) -> ()
        n194 = local write "LedVerdeD2"(FALSE ("LedVerdeD1")) -> ()
        n195 = local write "LedRojoD2"(TRUE ("LedRojoD1")) -> ()
        n196 = call-poly "Enqueue Message.vi"("error in (no error)"=w461, "Message"="Cumplimiento", "Message Queue"=w459) -> ("error out"=w449:errorcluster)  [unwired: 7 in, 1 out]
        n197 = local write "1_D2"(w462) -> ()
        n198 = local write "2_D2"(w462) -> ()
        n199 = local write "3_D2"(w462) -> ()
        n200 = Unbundle By Name(w450) -> ("Control references"=w452:T2)
        n201 = call-poly "get control reference by name.vi"("error in (no error)"=w449, "Control name"="Capturar_D2", "Control references"=w452) -> ("error out"=w453:errorcluster, "Ctl Refnum"=w456:refnum<vi>)  [unwired: 3 in]
        n202 = Build Array(w456) -> (w455:refnum<vi>[])
        n203 = call "Enable_Visible Buttons.vi"("Enable? (T)"=FALSE, "Controls Ref Array"=w455) -> ()  [unwired: 10 in]
        n204 = call-poly "get control reference by name.vi"("error in (no error)"=w453, "Control name"="CapturaGlobal_D2", "Control references"=w452) -> ("error out"=w445:errorcluster, "Ctl Refnum"=w454:refnum<vi>)  [unwired: 3 in]
        n205 = Build Array(w454) -> (w448:refnum<vi>[])
        n206 = call "Enable_Visible Buttons.vi"("Enable? (T)"=TRUE, "Controls Ref Array"=w448) -> ()  [unwired: 10 in]
        n207 = call "FGV_timer.vi"("error in (no error)"=w445, "time target"=w443, "action"=enum16{"get time", "start timer"}."start timer") -> ("error out"=w444:errorcluster)  [unwired: 2 out]
      }
      frame "---- Evaluacion ----" {
      }
      frame "Cumplimiento" {
        # "TD"
        # "Frecuencia"
        # "NPS"
        n208 = call "CumplimientoNPS.vi"("error in (no error)"=w478, "Prueba21 in"=w476) -> ("error out"=w477:errorcluster, "Prueba21 out"=w474:refnum<class "Prueba21.lvclass">)  [unwired: 8 in]
        n209 = call "CumplimientoFrecuencia.vi"("error in (no error)"=w477, "Prueba21_1 in"=w474) -> ("error out"=w475:errorcluster, "Prueba21_1 out"=w472:refnum<class "Prueba21.lvclass">)  [unwired: 8 in]
        n210 = call "CumplimientoTD.vi"("error in (no error)"=w475, "Prueba21_1 in"=w472) -> ("error out"=w473:errorcluster, "Prueba21_1 out"=w471:refnum<class "Prueba21.lvclass">)  [unwired: 8 in]
        n211 = call-poly "Enqueue Message.vi"("error in (no error)"=w473, "Message"="Listo_Evaluar?", "Message Queue"=w469) -> ("error out"=w470:errorcluster)  [unwired: 7 in, 1 out]
      }
      frame "Listo_Evaluar?" {
        n212 = call "ListoEvaluar.vi"("error in (no error)"=w486, "Prueba21 in"=w484) -> ("error out"=w485:errorcluster, "listo_para_evaluar"=w479:bool, "Prueba21 out"=w483:refnum<class "Prueba21.lvclass">)  [unwired: 7 in]
        n213 = Unbundle By Name(w481) -> ("MHL"=w480:refnum<queue>)
        n214 = case shown="True" w479 {
          tunnel: w485 -> [w487 w491]
          tunnel: [w487 w490] -> w482
          tunnel: w480 -> [_ w489]
          frame False {
          }
          frame True {
            n215 = call-poly "Enqueue Message.vi"("error in (no error)"=w491, "Message"="Evaluar", "Message Queue"=w489) -> ("error out"=w490:errorcluster)  [unwired: 7 in, 1 out]
          }
        }
      }
      frame "Evaluar" {
        n216 = call "Evaluar.vi"("error in (no error)"=w500, "Prueba21_1 in"=w498) -> ("error out"=w499:errorcluster, "pasa?"=w492:bool, "Prueba21_1 out"=w497:refnum<class "Prueba21.lvclass">)  [unwired: 7 in]
        "cumple" <- w492
        n217 = Not(x=w492) -> (.not. x?=→"no_cumple":bool)
        n218 = Select(t="Cumple", s=w492, f="No Cumple") -> (s? t:f=→"Resultado":string)
      }
      frame "--------------------------Contoles---------------------------" {
      }
    }
    n219 = call "Error Handler - Message Handling Loop.vi"("error in (no error)"=w48, "Message Queue"=w49) -> ("dup error in"=w47:errorcluster)  [unwired: 8 in, 1 out]
  }
  "Prueba21 out" <- w26
  n220 = call "Inst_CNT90.vi"("error in"=w14, "All Message Queues in"=w15, "Prueba21_1 in"=w10) -> ("error out"=w22:errorcluster)  [unwired: 8 in]
  n221 = call "Inst_K2002.vi"("error in"=w14, "All Message Queues in"=w15, "Prueba31 in"=w10) -> ("error out"=w21:errorcluster)  [unwired: 8 in]
  n222 = while {
    tunnel: w30 -> [w511]
    tunnel: [w507] -> w33
    shift-right: [w509] -> w32
    shift-left: w34 -> [w510]
    stop <- w503 stop-if-true
    # "Event Handling Loop"
    n223 = event shown="[2] \"salir\": Value Change" {
      selector: w510 -> [_ _ _ _ _ _ _ _ _ _ _]
      dyn-events: [_ _ _ _ _ _ _ _ _ _ _] -> w509
      timeout: _ -> [_ _ _ _ _ _ _ _ _ _ _]
      tunnel: w511 -> [w514 _ w525 w533 w539 w542 w545 w548 w551 w554 w560]
      tunnel: [w516 _ w527 w534 w540 w543 w546 w549 w552 w555 w561] -> w508
      tunnel: [w515 _ _ _ _ _ _ _ _ _ _] -> w506
      tunnel: [_ w517 _ _ _ _ _ _ _ _ _] -> w504
      event Panel Close? {
        w512 = TRUE
        n224 = event-data() -> ()  [unwired: 1 in, 1 out]
        n225 = call-poly "Enqueue Message.vi"("Priority Message? (F)"=w512, "Message"="Confirmar Salida", "Message Queue"=w514) -> ("error out"=w516:errorcluster, "dup Message Queue"=w515:refnum<queue>)  [unwired: 7 in]
        n226 = event-data("Discard?"=w512) -> ()  [unwired: 1 in, 1 out]
      }
      event User Event {
        n227 = event-data() -> ("User Event"=w519:string, "Event Data"=w518:variant)  [unwired: 1 in]
        n228 = case shown="\"Exit EHL\"" w519 {
          tunnel: w518 -> [_ w521]
          tunnel: [_ w520] -> w517
          frame Default {
          }
          frame "Exit EHL" {
            # "#evangelio Termina\nla ejecucion del EHL"
            n229 = Variant To Data(type=TRUE, Variant=w521) -> (data=w520:bool)  [unwired: 1 in, 1 out]
          }
        }
      }
      event "salir": Value Change {
        n230 = event-data() -> ()  [unwired: 1 in, 1 out]
        n231 = call-poly "Enqueue Message.vi"("Message"="Detener_Instrumento", "Message Queue"=w525) -> ("dup Message Queue"=w524:refnum<queue>)  [unwired: 8 in, 1 out]
        n232 = call-poly "Enqueue Message.vi"("Message"="Exit", "Message Queue"=w524) -> ("error out"=w527:errorcluster)  [unwired: 8 in, 1 out]
      }
      event "CapturaGlobal_D1": Value Change {
        n233 = event-data() -> ()  [unwired: 1 in, 1 out]
        n234 = Select(t="IniciarDAQ" ("Message"), s="CapturaGlobal_D1", f="DetenerDAQ" ("Message")) -> (s? t:f=w529:string)
        n235 = call-poly "Enqueue Message.vi"("Priority Message? (F)"=TRUE, "Message"=w529, "Message Queue"=w533) -> ("error out"=w534:errorcluster)  [unwired: 7 in, 1 out]
      }
      event "CapturaGlobal_D2": Value Change {
        n236 = event-data() -> ()  [unwired: 1 in, 1 out]
        n237 = Select(t="IniciarDAQ" ("Message"), s="CapturaGlobal_D2", f="DetenerDAQ" ("Message")) -> (s? t:f=w536:string)
        n238 = call-poly "Enqueue Message.vi"("Message"=w536, "Message Queue"=w539) -> ("error out"=w540:errorcluster)  [unwired: 8 in, 1 out]
      }
      event "1_D1", "2_D1", "3_D1": Value Change {
        n239 = event-data() -> ()  [unwired: 1 in, 1 out]
        n240 = call-poly "Enqueue Message.vi"("Message"="HabilitarCaptura1", "Message Queue"=w542) -> ("error out"=w543:errorcluster)  [unwired: 8 in, 1 out]
      }
      event "1_D2", "2_D2", "3_D2": Value Change {
        n241 = event-data() -> ()  [unwired: 1 in, 1 out]
        n242 = call-poly "Enqueue Message.vi"("Message"="HabilitarCaptura2", "Message Queue"=w545) -> ("error out"=w546:errorcluster)  [unwired: 8 in, 1 out]
      }
      event "Capturar_D1": Value Change {
        n243 = event-data() -> ()  [unwired: 1 in, 1 out]
        n244 = call-poly "Enqueue Message.vi"("Message"="IniciarCaptura1", "Message Queue"=w548) -> ("error out"=w549:errorcluster)  [unwired: 8 in, 1 out]
      }
      event "Capturar_D2": Value Change {
        n245 = event-data() -> ()  [unwired: 1 in, 1 out]
        n246 = call-poly "Enqueue Message.vi"("Message"="IniciarCaptura2", "Message Queue"=w551) -> ("error out"=w552:errorcluster)  [unwired: 8 in, 1 out]
      }
      event "seguir_D2": Value Change {
        n247 = event-data() -> ()  [unwired: 1 in, 1 out]
        n248 = call-poly "Enqueue Message.vi"("Message"="SeguirD2", "Message Queue"=w554) -> ("error out"=w555:errorcluster)  [unwired: 8 in, 1 out]
      }
      event "generar_ext": Value Change {
        n249 = event-data() -> ()  [unwired: 1 in, 1 out]
        n250 = Select(t="IniciarGEN_Ext" ("Message"), s="generar_ext", f="DetenerGEN_Ext" ("Message")) -> (s? t:f=w557:string)
        n251 = call-poly "Enqueue Message.vi"("Message"=w557, "Message Queue"=w560) -> ("error out"=w561:errorcluster)  [unwired: 8 in, 1 out]
      }
    }
    n252 = call "Error Handler - Event Handling Loop.vi"("error in (no error)"=w508, "Message Queue"=w506) -> ("dup error in"=w507:errorcluster, "Error?"=w505:bool)  [unwired: 7 in, 1 out]
    n253 = Or(x=w504, y=w505) -> (x .or. y?=w503:bool)
  }
  n254 = Unregister For Events(event registration refnum=w32, error in=w33) -> (error out=w29:errorcluster)
  n255 = Merge Errors(w29, w28, w22, w21, w13) -> (w27:errorcluster)
  n256 = call "Destroy User Event - Stop.vi"("error in (no error)"=w27, "User Event"=w25) -> ("error out"=→"error out":errorcluster)  [unwired: 9 in]
